vi "Msgbox UI.vi"(5 "Show Cancel (Default - False)":bool, 8 "Error In":errorcluster, 9 "<xxxxxx> + Pre+Description+Post (Unicode)":string, 10 "[ShortDescription] (Unicode)":string, 11 "[MessageType]":string) -> (0 "Error Out":errorcluster, 1 "{OK} / {Cancel} Click String":string, 3 "OK Out":bool caption="OK1")   [LabVIEW 2020]
uses:
  <vilib>/Utility/miscctls.llb/LVPointTypeDef.ctl
panel:
  out "Ref error out":errorcluster
  out "[ShortDescription]":string
  out "Ring":u16(ring)
  out "Message Display":string
  in  "Cancel":bool caption="OK1"
  in  "OK":bool caption="OK1"
  # "Additional Info."
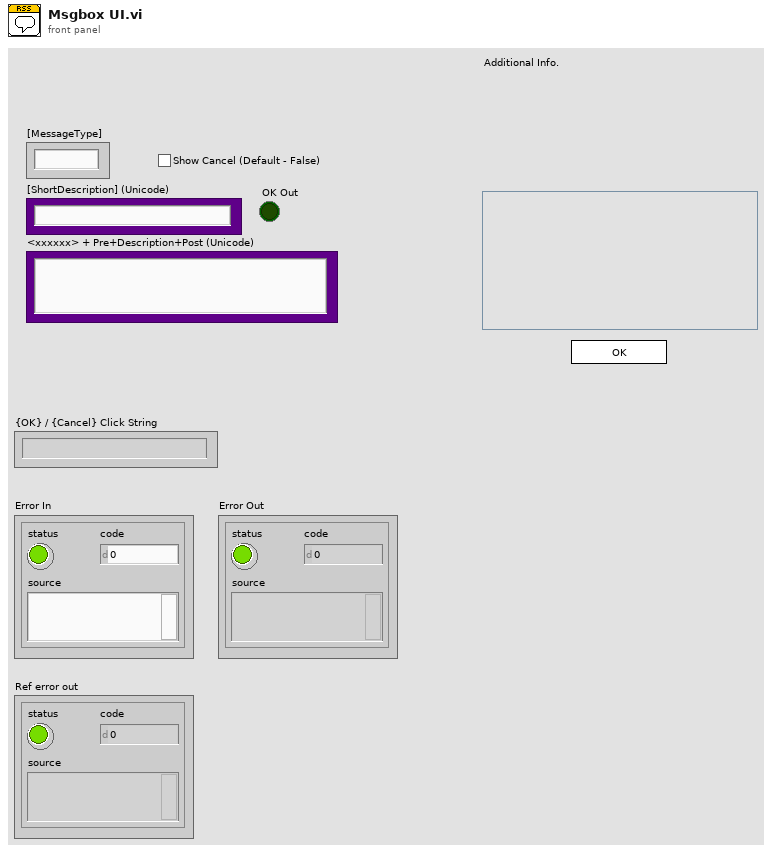
[diagram p1: front panel]
types:
  T1 = typedef "LVPointTypeDef.ctl" = cluster{"Horizontal":i16, "Vertical":i16}
  T2 = enum32{"Invalid", "Standard", "Closed", "Hidden", "Minimized", "Maximized"}
  T3 = typedef "Enum - InteractiveMode-SubVIMode.ctl" = enum16{"Interactive", "subVI Mode"}
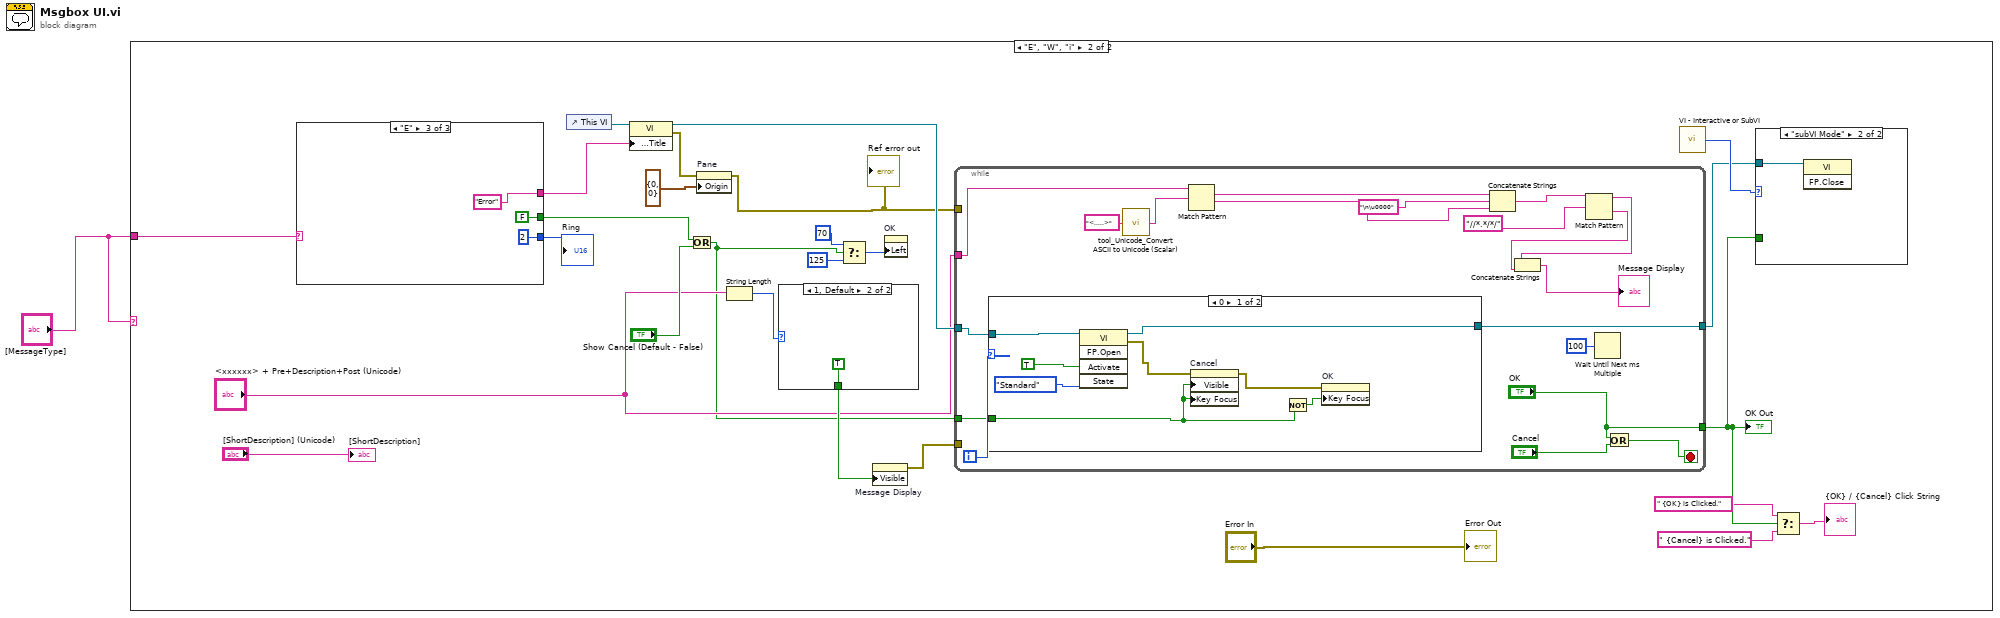
[diagram p0: block diagram]
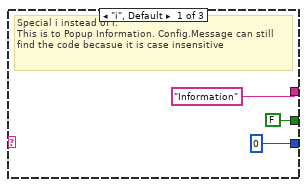
[diagram p3: hidden frame]
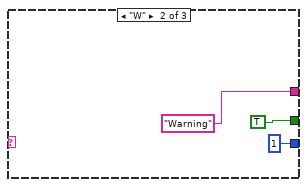
[diagram p4: hidden frame]
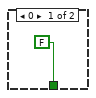
[diagram p6: hidden frame]
diagram:
  n1 = case shown="\"E\", \"W\", \"i\"" "[MessageType]" {
    tunnel: "[MessageType]" -> [_ w5]
    frame "I", Default {
      # "No Popup for Information"
    }
    frame "E", "W", "i" {
      n2 = case shown="\"E\"" w5 {
        tunnel: [u16 0 u16 1 u16 2] -> w18
        tunnel: ["Information" "Warning" "Error"] -> w17
        tunnel: [FALSE TRUE FALSE] -> w6
        frame "i", Default {
          # "Special i instead of I.\nThis is to Popup Information. Config.Message can still\nfind the code becasue it is case insensitive"
        }
        frame "W" {
        }
        frame "E" {
        }
      }
      "Ring" <- w18
      n3 = control-ref of="This VI"() -> (w27:refnum<vi>)
      n4 = property class="VI"(reference=w27, "Front Panel.Title"=w17) -> (reference out=w10:refnum<vi>, error out=w11:errorcluster)  [unwired: 1 in]
      n5 = Or(x=w6, y="Show Cancel (Default - False)") -> (x .or. y?=w2:bool)
      n6 = property on="Pane" class="Pane"(error in=w11, "Origin"=T1 {"Horizontal"=0, "Vertical"=0}) -> (error out=w8:errorcluster)  [unwired: 1 in, 1 out]
      "Ref error out" <- w8
      n7 = String Length(string="<xxxxxx> + Pre+Description+Post (Unicode)") -> (length=w26:i32)
      n8 = case shown="1, Default" w26 {
        tunnel: [FALSE ("Visible") TRUE ("Visible")] -> w25
        frame 0 {
        }
        frame 1, Default {
        }
      }
      n9 = Select(t=70, s=w2, f=125) -> (s? t:f=w21:i32)
      n10 = property on="Message Display" class="Str"("Visible"=w25) -> (error out=w24:errorcluster)  [unwired: 2 in, 1 out]
      n11 = property on="OK" class="Bool"("Left"=w21) -> ()  [unwired: 2 in, 2 out]
      n12 = while {
        tunnel: "<xxxxxx> + Pre+Description+Post (Unicode)" -> [w50]
        tunnel: ["OK"] -> w16
        tunnel: w24 -> [_]
        tunnel: w8 -> [_]
        tunnel: w10 -> [w46]
        tunnel: [w45] -> w9
        tunnel: w2 -> [w44]
        i -> [w47]
        stop <- w57 stop-if-true
        n13 = case shown="0" w47 {
          tunnel: w46 -> [w66 w67]
          tunnel: [w65 w67] -> w45
          tunnel: w44 -> [w60 _]
          frame 0 {
            n14 = invoke class="VI" method="FP.Open"(reference=w66, "Activate"=TRUE ("Activate?"), "State"=T2."Standard") -> (reference out=w65:refnum<vi>, error out=w62:errorcluster)  [unwired: 2 in, 3 out]
            n15 = property on="Cancel" class="Bool"(error in=w62, "Visible"=w60, "Key Focus"=w60) -> (error out=w59:errorcluster)  [unwired: 1 in, 1 out]
            n16 = Not(x=w60) -> (.not. x?=w61:bool)
            n17 = property on="OK" class="Bool"(error in=w59, "Key Focus"=w61) -> ()  [unwired: 1 in, 2 out]
          }
          frame 1, Default {
          }
        }
        n18 = call "tool_Unicode_Convert ASCII to Unicode (Scalar).vi"("ASCII"="<.....>") -> ("Unicode"=w42:string)  [unwired: 4 in]
        n19 = Match Pattern(string=w50, regular expression=w42) -> (match substring=w48:string, after substring=w41:string)  [unwired: 1 in, 2 out]
        n20 = Concatenate Strings(w48, "\n\u0000" ("string"), w41) -> (w49:string)
        n21 = Match Pattern(string=w49, regular expression="//*.*/*/") -> (before substring=w52:string, after substring=w51:string)  [unwired: 1 in, 2 out]
        n22 = Concatenate Strings(w52, w51) -> (→"Message Display":string)
        n23 = Wait Until Next ms Multiple(millisecond multiple=u32 100) -> ()  [unwired: 1 out]
        n24 = Or(x="OK", y="Cancel") -> (x .or. y?=w57:bool)
      }
      "OK Out" <- w16
      n25 = call "VI - Interactive or SubVI.vi"() -> ("Mode"=w22:T3)  [unwired: 5 in]
      n26 = case shown="\"subVI Mode\"" w22 {
        tunnel: w9 -> [_ w37]
        tunnel: w16 -> [_ _]
        frame "Interactive", Default {
          # "Leave it OPEN"
        }
        frame "subVI Mode" {
          n27 = invoke class="VI" method="FP.Close"(reference=w37) -> ()  [unwired: 2 in, 3 out]
        }
      }
      n28 = Select(t=" {OK} is Clicked.", s=w16, f=" {Cancel} is Clicked.") -> (s? t:f=→"{OK} / {Cancel} Click String":string)
      "[ShortDescription]" <- "[ShortDescription] (Unicode)"
      "Error Out" <- "Error In"
    }
  }
